vi "Temp1.vi"(7 "error in":errorcluster) -> (27 "error out":errorcluster)   [LabVIEW 2015]
uses:
  <vilib>/vision/NI_Vision_Development_Module.lvlib
panel:
  out "Image Out":T1(plugin-control)
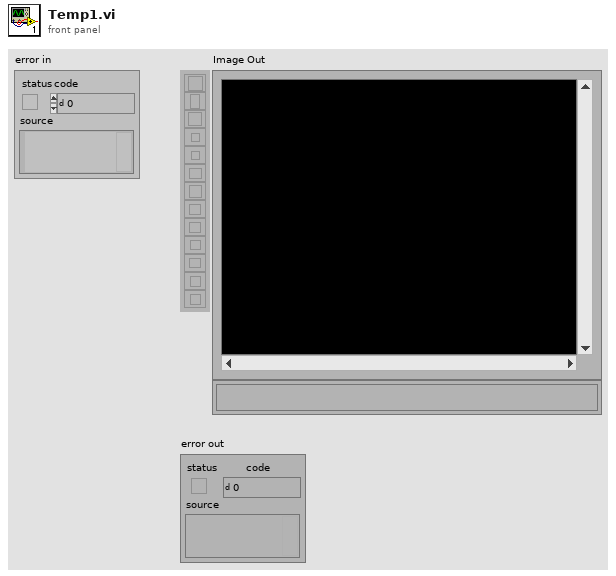
[diagram p1: front panel]
types:
  T1 = typedef "IMAQ Image.ctl" = refnum<image>
  T2 = cluster{"Feature":u32, "Points IDs":cluster{"GUID":string, "Index":i32}[]}[]
  T3 = cluster{"Number of Matches Requested":i32, "Minimum Match Score":sgl, "Angle Ranges":cluster{"Start Angle":sgl, "End Angle":sgl}[]}
  T4 = cluster{"Global Rectangle":i32[], "Contours":cluster{"ID":enum32{"External", "Internal"}, "Type":u32, "Coordinates":i32[]}[]}
  T5 = cluster{"Origin Pixel":cluster{"X":sgl, "Y":sgl}, "X Axis Pixel":cluster{"X":sgl, "Y":sgl}, "Axis Reference":u32}
  T6 = typedef "Image Type" = u32
  T7 = cluster{"Position":cluster{"x":sgl, "y":sgl}, "Angle":sgl, "Scale":sgl, "Score":sgl, "Bounding Box":cluster{"x":sgl, "y":sgl}[]}[]
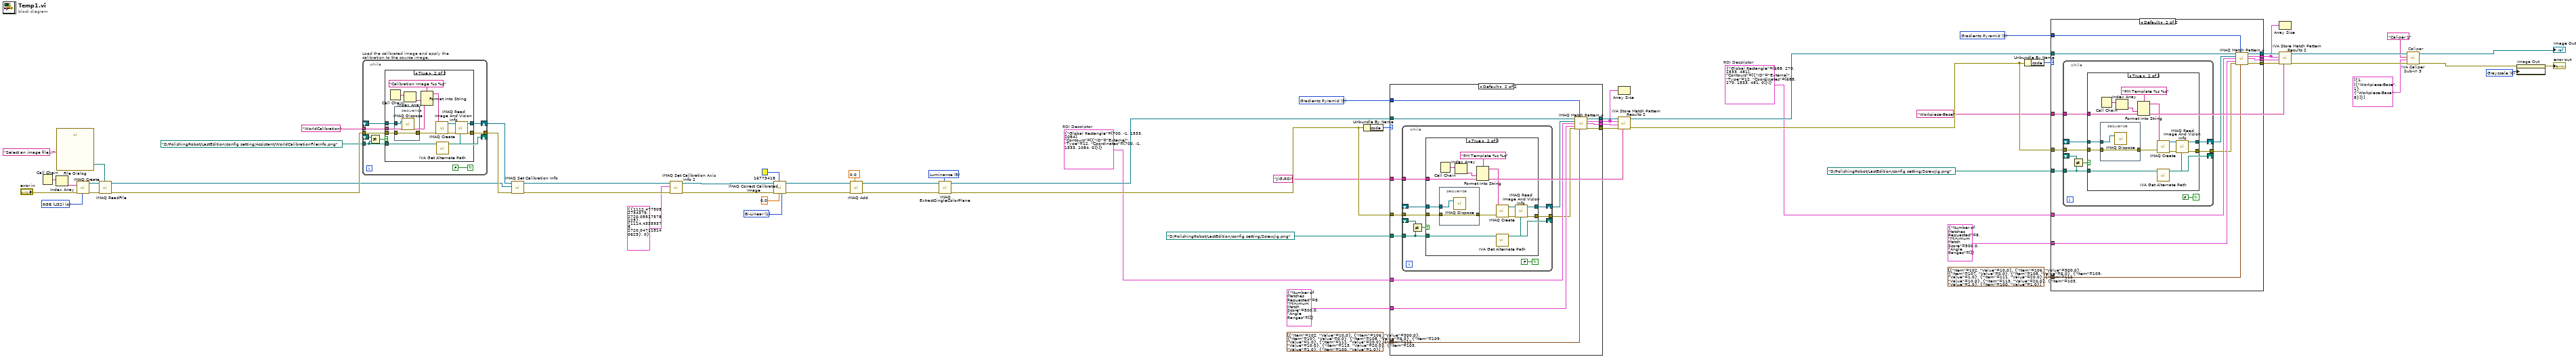
[diagram p0: block diagram]
diagram:
  w1 = u32 0 items=["Grayscale", "Binary", "Gradient", "Rainbow", "Temperature", "User Defined", "Binary 16 Bit", "Gradient 16 Bit", "Rainbow 16 Bit", "Temperature 16 Bit", "User Defined 16 Bit"] ("Palette Type")
  w14 = 3 items=["All", "Low Discrepancy Sampling", "Grayscale Value Pyramid", "Gradients Pyramid"] ("Algorithm")
  w10 = "Workpiece-Base" ("Step Name")
  w13 = T4 {"Global Rectangle"=[688, 270, 1533, 481], "Contours"=[{"ID"=enum."External", "Type"=12, "Coordinates"=[688, 270, 1533, 481, 0]}]}  # ROI Descriptor
  w27 = 3 items=["All", "Low Discrepancy Sampling", "Grayscale Value Pyramid", "Gradients Pyramid"] ("Algorithm")
  w23 = "JiG-ROI" ("Step Name")
  w26 = T4 {"Global Rectangle"=[700, -1, 1533, 1084], "Contours"=[{"ID"=enum."External", "Type"=12, "Coordinates"=[700, -1, 1533, 1084, 0]}]}  # ROI Descriptor
  w36 = 5 items=["Red", "Green", "Blue", "Hue", "Saturation", "Luminance", "Value", "Intensity"] ("Color Plane")
  w44 = u32 1 items=["Zero Order", "Bi-Linear", "Quadratic", "Cubic Spline"] ("Interpolation Type")
  w54 = T6 4 items=["Grayscale (U8)", "Grayscale (I16)", "Grayscale (SGL)", "Complex (CSG)", "RGB (U32)", "HSL (U32)", "RGB (U64)", "Grayscale (U16)"] ("Image Type")
  # "Caliper"
  n1 = Call Chain() -> (call chain=w58:string[])
  n2 = Index Array(array=w58) -> (element=w57:string)  [unwired: 1 in]
  n3 = call "File Dialog"("prompt"="Select an image file...") -> ("selected path"=w55:path)  [unwired: 6 in, 8 out]
  n4 = call "IMAQ Create"("Image Name"=w57, "Image Type"=w54, "error in (no error)"="error in") -> ("New Image"=w61:T1, "error out"=w60:errorcluster)  [unwired: 1 in, 1 out]
  n5 = call "IMAQ ReadFile"("File Path"=w55, "error in (no error)"=w60, "Image"=w61) -> ("error out"=w62:errorcluster, "Image Out"=w49:T1)  [unwired: 2 in, 5 out]
  n6 = while "Load the calibrated image and apply the calibration to the source image." {
    shift-right: [w71] -> w52
    shift-left: _ -> [w70]
    tunnel: [w68] -> w51
    tunnel: w62 -> [w67]
    tunnel: path "D:/PolishingRobot/LastEdition/config setting/Assistant/WorldCalibrationFileInfo.png" ("File Path") -> [w63]
    tunnel: "WorldCalibration" ("Step Name") -> [w66]
    shift-right: [w63] -> _
    shift-left: _ -> [w65]
    stop <- FALSE continue-if-true
    n7 = Not Equal?(x=w65, y=w63) -> (x != y?=w64:bool)
    n8 = case shown="True" w64 {
      tunnel: [w73 w85] -> w71
      tunnel: w70 -> [w73 w77]
      tunnel: [w72 w82] -> w68
      tunnel: w67 -> [w72 w78]
      tunnel: w63 -> [_ w75]
      tunnel: w66 -> [_ w79]
      frame False {
      }
      frame True {
        n9 = Call Chain() -> (call chain=w81:string[])
        n10 = stacked-sequence {
          tunnel: w78 -> [w88]
          tunnel: w77 -> [w89]
          tunnel: [w88] -> w76
          frame #0 {
            n11 = call "IMAQ Dispose"("Image"=w89) -> ()  [unwired: 2 in, 4 out]
          }
        }
        n12 = Index Array(array=w81) -> (element=w80:string)  [unwired: 1 in]
        n13 = Format Into String(format string="Calibration Image %s %s" ("Image Name"), w80, w79) -> (resulting string=w87:string)  [unwired: 2 in, 1 out]
        n14 = call "IMAQ Create"("Image Name"=w87, "error in (no error)"=w76) -> ("New Image"=w84:T1, "error out"=w83:errorcluster)  [unwired: 2 in, 1 out]
        n15 = call <vilib>:"IVA Get Alternate Path.vi"("Path In"=w75) -> ("Path Out"=w74:path)  [unwired: 10 out]
        n16 = call "IMAQ Read Image And Vision Info"("File Path"=w74, "error in (no error)"=w83, "Image"=w84) -> ("error out"=w82:errorcluster, "Image Out"=w85:T1)  [unwired: 1 in, 6 out]
      }
    }
  }
  n17 = call "IMAQ Set Calibration Info"("error in (no error)"=w51, "Image Dst"=w49, "Image Src"=w52) -> ("error out"=w50:errorcluster, "Calibrated Image"=w46:T1)  [unwired: 1 in, 6 out]
  n18 = call-poly "IMAQ Set Calibration Axis Info 2"("error in (no error)"=w50, "Calibration Axis Info"=T5 {"Origin Pixel"={"X"=1112.4779, "Y"=2720.0552}, "X Axis Pixel"={"X"=1114.4336, "Y"=2720.047}, "Axis Reference"=0}, "Calibration Template Image In"=w46) -> ("error out"=w47:errorcluster, "Calibration Template Image Out"=w42:T1)  [unwired: 7 out]
  n19 = call "IMAQ Correct Calibrated Image"("Interpolation Type"=w44, "Replace Value"=sgl 0.0, "Color Replace Value"=u32 16773418, "error in (no error)"=w47, "Image Src"=w42) -> ("error out"=w43:errorcluster, "Corrected Image"=w38:T1)  [unwired: 2 in, 3 out]
  n20 = call "IMAQ Add"("Image Src A"=w38, "Constant"=sgl 0.0, "error in (no error)"=w43) -> ("Image Dst Out"=w35:T1, "error out"=w37:errorcluster)  [unwired: 2 in, 2 out]
  n21 = call "IMAQ ExtractSingleColorPlane"("Color Plane"=w36, "error in (no error)"=w37, "Image Src"=w35) -> ("error out"=w34:errorcluster, "Image Dst Out"=w32:T1)  [unwired: 1 in, 6 out]
  n22 = Unbundle By Name(w34) -> ("code"=w28:i32)
  n23 = case shown="Default" w28 {
    tunnel: path "D:/PolishingRobot/LastEdition/config setting/ScrewJig.png" ("Template File Path") -> [_ w104]
    tunnel: w34 -> [_ w103]
    tunnel: w32 -> [w90 w98]
    tunnel: [_ w99] -> w31
    tunnel: [_ w100] -> w22
    tunnel: [w90 w97] -> w29
    tunnel: w23 -> [_ w102]
    tunnel: w27 -> [_ w96]
    tunnel: w26 -> [_ w95]
    tunnel: T3 {"Number of Matches Requested"=8, "Minimum Match Score"=500.0, "Angle Ranges"=[]} ("Parameters") -> [_ w94]
    tunnel: cluster{"Item":u16, "Value":dbl}[] [{"Item"=102, "Value"=10.0}, {"Item"=106, "Value"=300.0}, {"Item"=107, "Value"=0.0}, {"Item"=108, "Value"=6.0}, {"Item"=109, "Value"=1.0}, {"Item"=111, "Value"=20.0}, {"Item"=112, "Value"=10.0}, {"Item"=113, "Value"=20.0}, {"Item"=103, "Value"=1.0}, {"Item"=100, "Value"=1.0}] ("Advanced Options") -> [_ w92]
    tunnel: [_ w91] -> w21
    frame -1074396199, -1074396198 {
      # "Discard Coordinate System Error"
    }
    frame Default {
      n24 = while {
        shift-right: [w113] -> w101
        shift-left: _ -> [w112]
        tunnel: [w110] -> w93
        tunnel: w103 -> [w109]
        tunnel: w104 -> [w106]
        tunnel: w102 -> [w108]
        shift-right: [w106] -> _
        shift-left: _ -> [w107]
        stop <- FALSE continue-if-true
        n25 = Not Equal?(x=w107, y=w106) -> (x != y?=w105:bool)
        n26 = case shown="True" w105 {
          tunnel: [w115 w127] -> w113
          tunnel: w112 -> [w115 w118]
          tunnel: [w114 w124] -> w110
          tunnel: w109 -> [w114 w117]
          tunnel: w106 -> [_ w120]
          tunnel: w108 -> [_ w121]
          frame False {
          }
          frame True {
            n27 = stacked-sequence {
              tunnel: w118 -> [w131]
              tunnel: w117 -> [w130]
              tunnel: [w130] -> w116
              frame #0 {
                n28 = call "IMAQ Dispose"("Image"=w131) -> ()  [unwired: 2 in, 4 out]
              }
            }
            n29 = Call Chain() -> (call chain=w123:string[])
            n30 = Index Array(array=w123) -> (element=w122:string)  [unwired: 1 in]
            n31 = Format Into String(format string="PM Template %s %s" ("Image Name"), w122, w121) -> (resulting string=w129:string)  [unwired: 2 in, 1 out]
            n32 = call "IMAQ Create"("Image Name"=w129, "error in (no error)"=w116) -> ("New Image"=w126:T1, "error out"=w125:errorcluster)  [unwired: 2 in, 1 out]
            n33 = call <vilib>:"IVA Get Alternate Path.vi"("Path In"=w120) -> ("Path Out"=w119:path)  [unwired: 10 out]
            n34 = call "IMAQ Read Image And Vision Info"("File Path"=w119, "error in (no error)"=w125, "Image"=w126) -> ("error out"=w124:errorcluster, "Image Out"=w127:T1)  [unwired: 1 in, 6 out]
          }
        }
      }
      n35 = call "IMAQ Match Pattern 4"("Image"=w98, "Algorithm"=w96, "Template Image"=w101, "ROI Descriptor"=w95, "Parameters"=w94, "error in (no error)"=w93, "Advanced Options"=w92) -> ("Image (duplicate)"=w97:T1, "Matches (pixel)"=w100:T7, "Matches (real-world)"=w91:T7, "error out"=w99:errorcluster)  [unwired: 4 in, 1 out]
    }
  }
  n36 = Array Size(array=w22) -> ()  [unwired: 1 out]
  n37 = call <vilib>:"IVA Store Match Pattern Results 2.vi"("Step Name"=w23, "error in (no error)"=w31, "Matches (real-world)"=w21, "Matches (pixel)"=w22, "Image in"=w29) -> ("error out"=w30:errorcluster, "Image dup"=w19:T1)  [unwired: 1 in, 4 out]
  n38 = Unbundle By Name(w30) -> ("code"=w15:i32)
  n39 = case shown="Default" w15 {
    tunnel: path "D:/PolishingRobot/LastEdition/config setting/ScrewJig.png" ("Template File Path") -> [_ w146]
    tunnel: w30 -> [_ w145]
    tunnel: w19 -> [w132 w140]
    tunnel: [_ w141] -> w18
    tunnel: [_ w142] -> w9
    tunnel: [w132 w139] -> w16
    tunnel: w10 -> [_ w144]
    tunnel: w14 -> [_ w138]
    tunnel: w13 -> [_ w137]
    tunnel: T3 {"Number of Matches Requested"=8, "Minimum Match Score"=500.0, "Angle Ranges"=[]} ("Parameters") -> [_ w136]
    tunnel: cluster{"Item":u16, "Value":dbl}[] [{"Item"=102, "Value"=10.0}, {"Item"=106, "Value"=300.0}, {"Item"=107, "Value"=0.0}, {"Item"=108, "Value"=6.0}, {"Item"=109, "Value"=1.0}, {"Item"=111, "Value"=20.0}, {"Item"=112, "Value"=10.0}, {"Item"=113, "Value"=20.0}, {"Item"=103, "Value"=1.0}, {"Item"=100, "Value"=1.0}] ("Advanced Options") -> [_ w134]
    tunnel: [_ w133] -> w8
    frame -1074396199, -1074396198 {
      # "Discard Coordinate System Error"
    }
    frame Default {
      n40 = while {
        shift-right: [w155] -> w143
        shift-left: _ -> [w154]
        tunnel: [w152] -> w135
        tunnel: w145 -> [w151]
        tunnel: w146 -> [w148]
        tunnel: w144 -> [w150]
        shift-right: [w148] -> _
        shift-left: _ -> [w149]
        stop <- FALSE continue-if-true
        n41 = Not Equal?(x=w149, y=w148) -> (x != y?=w147:bool)
        n42 = case shown="True" w147 {
          tunnel: [w157 w169] -> w155
          tunnel: w154 -> [w157 w160]
          tunnel: [w156 w166] -> w152
          tunnel: w151 -> [w156 w159]
          tunnel: w148 -> [_ w162]
          tunnel: w150 -> [_ w163]
          frame False {
          }
          frame True {
            n43 = stacked-sequence {
              tunnel: w160 -> [w173]
              tunnel: w159 -> [w172]
              tunnel: [w172] -> w158
              frame #0 {
                n44 = call "IMAQ Dispose"("Image"=w173) -> ()  [unwired: 2 in, 4 out]
              }
            }
            n45 = Call Chain() -> (call chain=w165:string[])
            n46 = Index Array(array=w165) -> (element=w164:string)  [unwired: 1 in]
            n47 = Format Into String(format string="PM Template %s %s" ("Image Name"), w164, w163) -> (resulting string=w171:string)  [unwired: 2 in, 1 out]
            n48 = call "IMAQ Create"("Image Name"=w171, "error in (no error)"=w158) -> ("New Image"=w168:T1, "error out"=w167:errorcluster)  [unwired: 2 in, 1 out]
            n49 = call <vilib>:"IVA Get Alternate Path.vi"("Path In"=w162) -> ("Path Out"=w161:path)  [unwired: 10 out]
            n50 = call "IMAQ Read Image And Vision Info"("File Path"=w161, "error in (no error)"=w167, "Image"=w168) -> ("error out"=w166:errorcluster, "Image Out"=w169:T1)  [unwired: 1 in, 6 out]
          }
        }
      }
      n51 = call "IMAQ Match Pattern 4"("Image"=w140, "Algorithm"=w138, "Template Image"=w143, "ROI Descriptor"=w137, "Parameters"=w136, "error in (no error)"=w135, "Advanced Options"=w134) -> ("Image (duplicate)"=w139:T1, "Matches (pixel)"=w142:T7, "Matches (real-world)"=w133:T7, "error out"=w141:errorcluster)  [unwired: 4 in, 1 out]
    }
  }
  n52 = Array Size(array=w9) -> ()  [unwired: 1 out]
  n53 = call <vilib>:"IVA Store Match Pattern Results 2.vi"("Step Name"=w10, "error in (no error)"=w18, "Matches (real-world)"=w8, "Matches (pixel)"=w9, "Image in"=w16) -> ("error out"=w17:errorcluster, "Image dup"=w7:T1)  [unwired: 1 in, 4 out]
  n54 = call <vilib>:"IVA Caliper Sub-VI 3.vi"("error in"=w17, "Parameters"=T2 [{"Feature"=1, "Points IDs"=[{"GUID"="Workpiece-Base", "Index"=1}, {"GUID"="Workpiece-Base", "Index"=8}]}], "Step Name"="Caliper 1", "Image In"=w7) -> ("error out"=w6:errorcluster, "Image Out"=→"Image Out":T1)  [unwired: 1 in, 5 out]
  n55 = property on="Image Out" class="ImageControl"(error in=w6, "Palette:Palette Type"=w1) -> (error out=→"error out":errorcluster)  [unwired: 1 in, 1 out]
